vi "Set Base Configuration.vi"(8 "error in (no error)":errorcluster, 11 "NI DMM Driver in":refnum<class "DMM.NI.lvclass">) -> (0 "error out":errorcluster, 3 "NI DMM Driver out":refnum<class "DMM.NI.lvclass">)   [LabVIEW 2020, in "NI DMM Driver.lvlib" / "DMM.NI.lvclass"]
doc: "Set the basic configuration on the instrument."
uses:
  DMM.NI.lvclass
  <instrlib>/niDMM/nidmm.llb/niDMM Powerline Frequency.ctl
  <instrlib>/niDMM/nidmm.llb/niDMM ADC Calibration.ctl
  <instrlib>/niDMM/nidmm.llb/niDMM Auto Zero.ctl
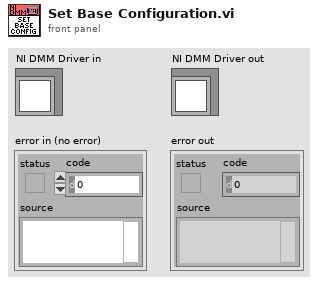
[diagram p1: front panel]
types:
  T1 = typedef "niDMM Powerline Frequency.ctl" = enum16{"60 Hz", "50 Hz"}
  T2 = typedef "niDMM Auto Zero.ctl" = i32
  T3 = typedef "niDMM ADC Calibration.ctl" = i32
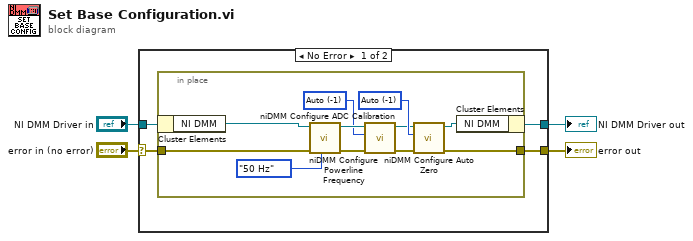
[diagram p0: block diagram]
diagram:
  n1 = case shown="No Error" "error in (no error)" {
    selector: "error in (no error)" -> [w7 w21]
    tunnel: [w6 w21] -> w3
    tunnel: [w5 w20] -> w2
    tunnel: "NI DMM Driver in" -> [w8 w20]
    frame No Error {
      n2 = in-place {
        in-place-border: w7 -> [w15]
        in-place-border: [w9] -> w6
        w14 = T2 -1 items=["Auto"=-1, "Off"=0, "On"=1, "Once"=2] ("Auto Zero")
        w16 = T3 -1 items=["Auto"=-1, "Off"=0, "On"=1] ("ADC Calibration")
        n3 = in-place-cluster #1(w8) -> ("NI DMM"=w19:refnum<k15>)
        n4 = call <instrlib>:"niDMM Configure Powerline Frequency.vi"("Powerline Frequency"=niDMM_Powerline_Frequency."50 Hz", "error in (no error)"=w15, "instrument handle"=w19) -> ("error out"=w11:errorcluster, "instrument handle out"=w18:refnum<k15>)  [unwired: 7 in]
        n5 = call <instrlib>:"niDMM Configure ADC Calibration.vi"("error in (no error)"=w11, "ADC Calibration"=w16, "instrument handle"=w18) -> ("error out"=w10:errorcluster, "instrument handle out"=w13:refnum<k15>)  [unwired: 7 in]
        n6 = call <instrlib>:"niDMM Configure Auto Zero.vi"("error in (no error)"=w10, "Auto Zero"=w14, "instrument handle"=w13) -> ("error out"=w9:errorcluster, "instrument handle out"=w12:refnum<k15>)  [unwired: 7 in]
        n7 = in-place-cluster #1("NI DMM"=w12) -> (w5:refnum<class "DMM.NI.lvclass">)
      }
    }
    frame Error {
    }
  }
  "error out" <- w3
  "NI DMM Driver out" <- w2
